vi "Rename Window.vi"(8 "error in (no error)":errorcluster, 9 "new window name (\"\")":string, 10 "current window name (\"\")":string, 11 "window refnum":T1) -> (0 "error out":errorcluster, 2 "prev window name":string, 3 "window refnum out":T1)   [LabVIEW 2020, in "MacroAssert.lvlib" / "Win Util.lvlib"]
doc: "This VI will rename the window identified either by its title or by its window refnum. If the window refnum is supplied, the name of the window before renaming is returned in the 'prev window name' output. If the window name is used to identify the window (current window name), then 'prev window name' = 'current window name'."
uses:
  Win Util.lvlib
  Window Refnum.ctl
  user32.dll
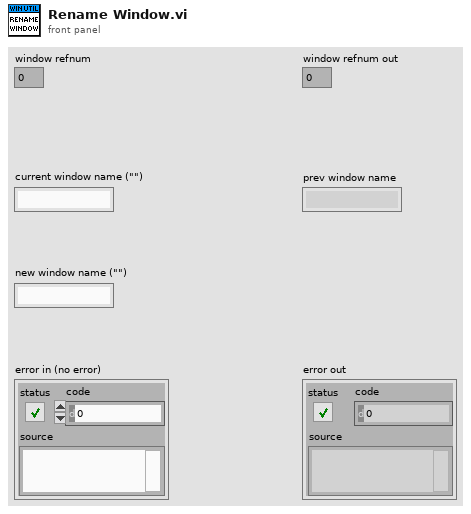
[diagram p1: front panel]
types:
  T1 = typedef "MacroAssert.lvlib/Win Util.lvlib/Window Refnum.ctl" = u64
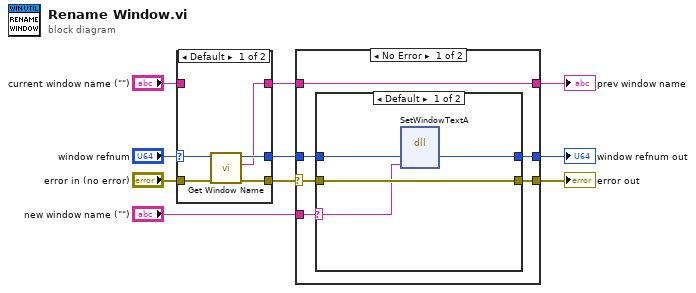
[diagram p0: block diagram]
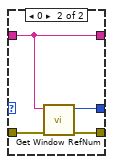
[diagram p2: hidden frame]
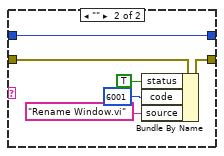
[diagram p3: hidden frame]
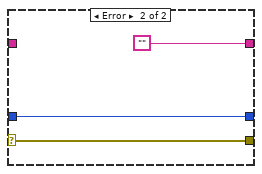
[diagram p4: hidden frame]
diagram:
  n1 = case shown="Default" "window refnum" {
    selector: "window refnum" -> [w15 _]
    tunnel: "error in (no error)" -> [w13 w19]
    tunnel: [w14 w18] -> w4
    tunnel: [w12 w17] -> w5
    tunnel: "current window name (\"\")" -> [_ w16]
    tunnel: [w11 w16] -> w3
    frame Default {
      n2 = call "Get Window Name.vi"("error in (no error)"=w13, "window refnum in"=w15) -> ("error out"=w12:errorcluster, "window name"=w11:string, "window refnum out"=w14:T1)  [unwired: 7 in]
    }
    frame 0 {
      n3 = call "Get Window RefNum.vi"("error in (no error)"=w19, "window name (\"\")"=w16) -> ("error out"=w17:errorcluster, "window refnum (NaWR)"=w18:T1)  [unwired: 6 out]
    }
  }
  n4 = case shown="No Error" w5 {
    selector: w5 -> [w21 w36]
    tunnel: w4 -> [w24 w37]
    tunnel: [w20 w37] -> w9
    tunnel: w3 -> [w25 _]
    tunnel: [w25 ""] -> w10
    tunnel: [w23 w36] -> w1
    tunnel: "new window name (\"\")" -> [w22 _]
    frame No Error {
      n5 = case shown="Default" w22 {
        selector: w22 -> [w26 _]
        tunnel: w24 -> [w28 w31]
        tunnel: [w29 w31] -> w20
        tunnel: [w27 w33] -> w23
        tunnel: w21 -> [w27 w32]
        frame Default {
          n6 = dll-call lib="USER32.DLL" fn="SetWindowTextA" label="SetWindowText"("hWnd"=w28, "windowName"=w26) -> ("hWnd"=w29:u64)  [unwired: 4 in, 3 out]
        }
        frame "" {
          n7 = Bundle By Name(cluster=w32, "status"=TRUE, "code"=6001, "source"="Rename Window.vi") -> (w33:errorcluster)
        }
      }
    }
    frame Error {
    }
  }
  "error out" <- w1
  "prev window name" <- w10
  "window refnum out" <- w9
